vi "LWXPS_XYZSplineParametersGet.vi"(0 "XPS Reference IN":refnum<k24>, 2 "XYZ group name":string, 5 "LabVIEW error IN":errorcluster) -> (12 "XPS Reference OUT":refnum<k24>, 13 "LabVIEW error OUT":errorcluster, 14 "Returned error code":i32, 15 "Trajectory file name":string, 16 "Velocity":dbl, 17 "Acceleration":dbl, 18 "Current element number":i32, 19 "XPS Error String":string)   [LabVIEW 2014]
uses:
  D:/XPSQ8_LabView_Library/Development/Source/Dll/Newport.XPS.CommandInterface.dll
  Dll/Newport.XPS.CommandInterface.dll
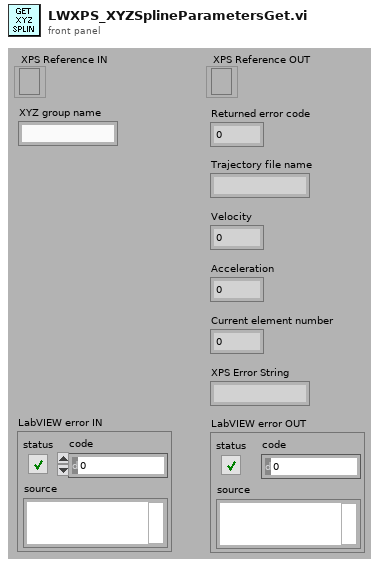
[diagram p1: front panel]
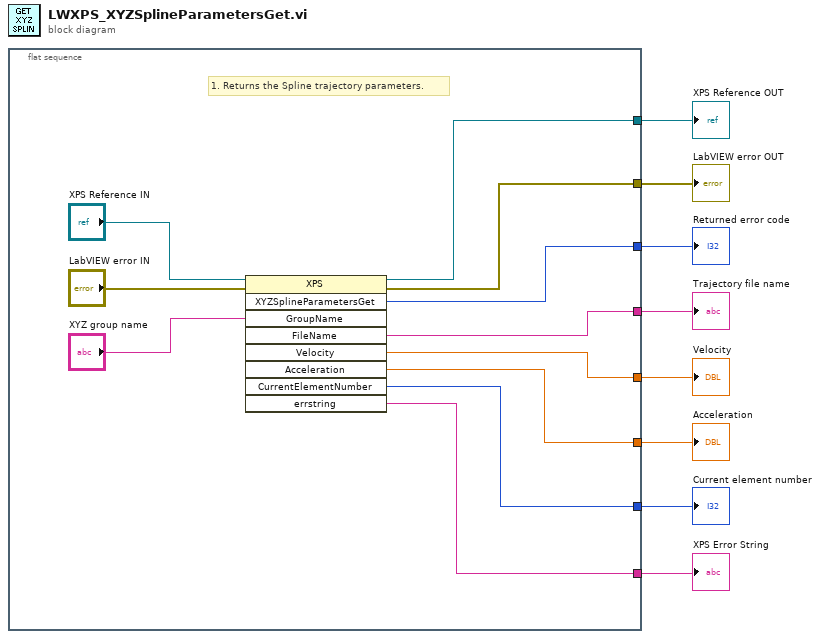
[diagram p0: block diagram]
diagram:
  n1 = flat-sequence {
    tunnel: [w17] -> w8
    tunnel: [w15] -> w7
    tunnel: [w18] -> w6
    tunnel: [w9] -> w2
    tunnel: [w14] -> w5
    tunnel: [w13] -> w3
    tunnel: [w12] -> w1
    tunnel: [w11] -> w4
    frame #0 {
      # "1. Returns the Spline trajectory parameters."
      n2 = invoke class="XPS" method="XYZSplineParametersGet"(reference="XPS Reference IN", error in="LabVIEW error IN", "GroupName"="XYZ group name") -> (reference out=w17:refnum<k24>, error out=w15:errorcluster, "XYZSplineParametersGet"=w18:i32, "FileName"=w9:string, "Velocity"=w14:dbl, "Acceleration"=w13:dbl, "CurrentElementNumber"=w12:i32, "errstring"=w11:string)  [unwired: 6 in, 1 out]
    }
  }
  "XPS Error String" <- w4
  "XPS Reference OUT" <- w8
  "LabVIEW error OUT" <- w7
  "Returned error code" <- w6
  "Velocity" <- w5
  "Acceleration" <- w3
  "Trajectory file name" <- w2
  "Current element number" <- w1
